vi "GetBarcode 1DResultNames.vi"(7 "ProjectName":string="Prj", 8 "error in (no error)":errorcluster, 10 "Analysis_Barcode 1D_Parameter":T2={"Barcode Search Options"={"Min Bar Width"=0.0, "Min Edge Strength"=0.0, "Min Bars"=0.0, "Skip Location Search?"=FALSE}, "Barcode Types To Search"=[enum."EAN 13", enum."Code 128", enum."Code 39"], "Barcode Grading Options"={"Calculate Grading Report"=FALSE, "Scan Width "=0.0}, "Number of Matches Requested"=1, "ROI"={"Global Rectangle"=[], "Contours"=[]}}, 11 "ROI_Name":string="ROI1") -> (0 "error out":errorcluster, 3 "ResultNames":string[](array[string]))   [LabVIEW 2019]
uses:
  Controls/Barcode 1D/Analysis_Barcode 1D_Parameter.ctl
  Controls/Barcode 1D/Analysis_Barcode 1D_Result.ctl
panel:
  out "Label.Text":string
  in  "Analysis_Barcode 1D_Result":T1 {"Barcodes"."Confidence Level" format="%.2f"; "Barcodes"."Barcode Type" items=["Reserved", "Codabar", "Code 39", "Code 93", "Code 128", "EAN 8", "EAN 13", "Interleaved 2 of 5", "MSI", "UPCA", "Pharmacode", "RSS Limited"]; "Barcodes"."Bounding Box"."y" format="%.2f"; "Barcodes"."Bounding Box"."x" format="%.2f"}
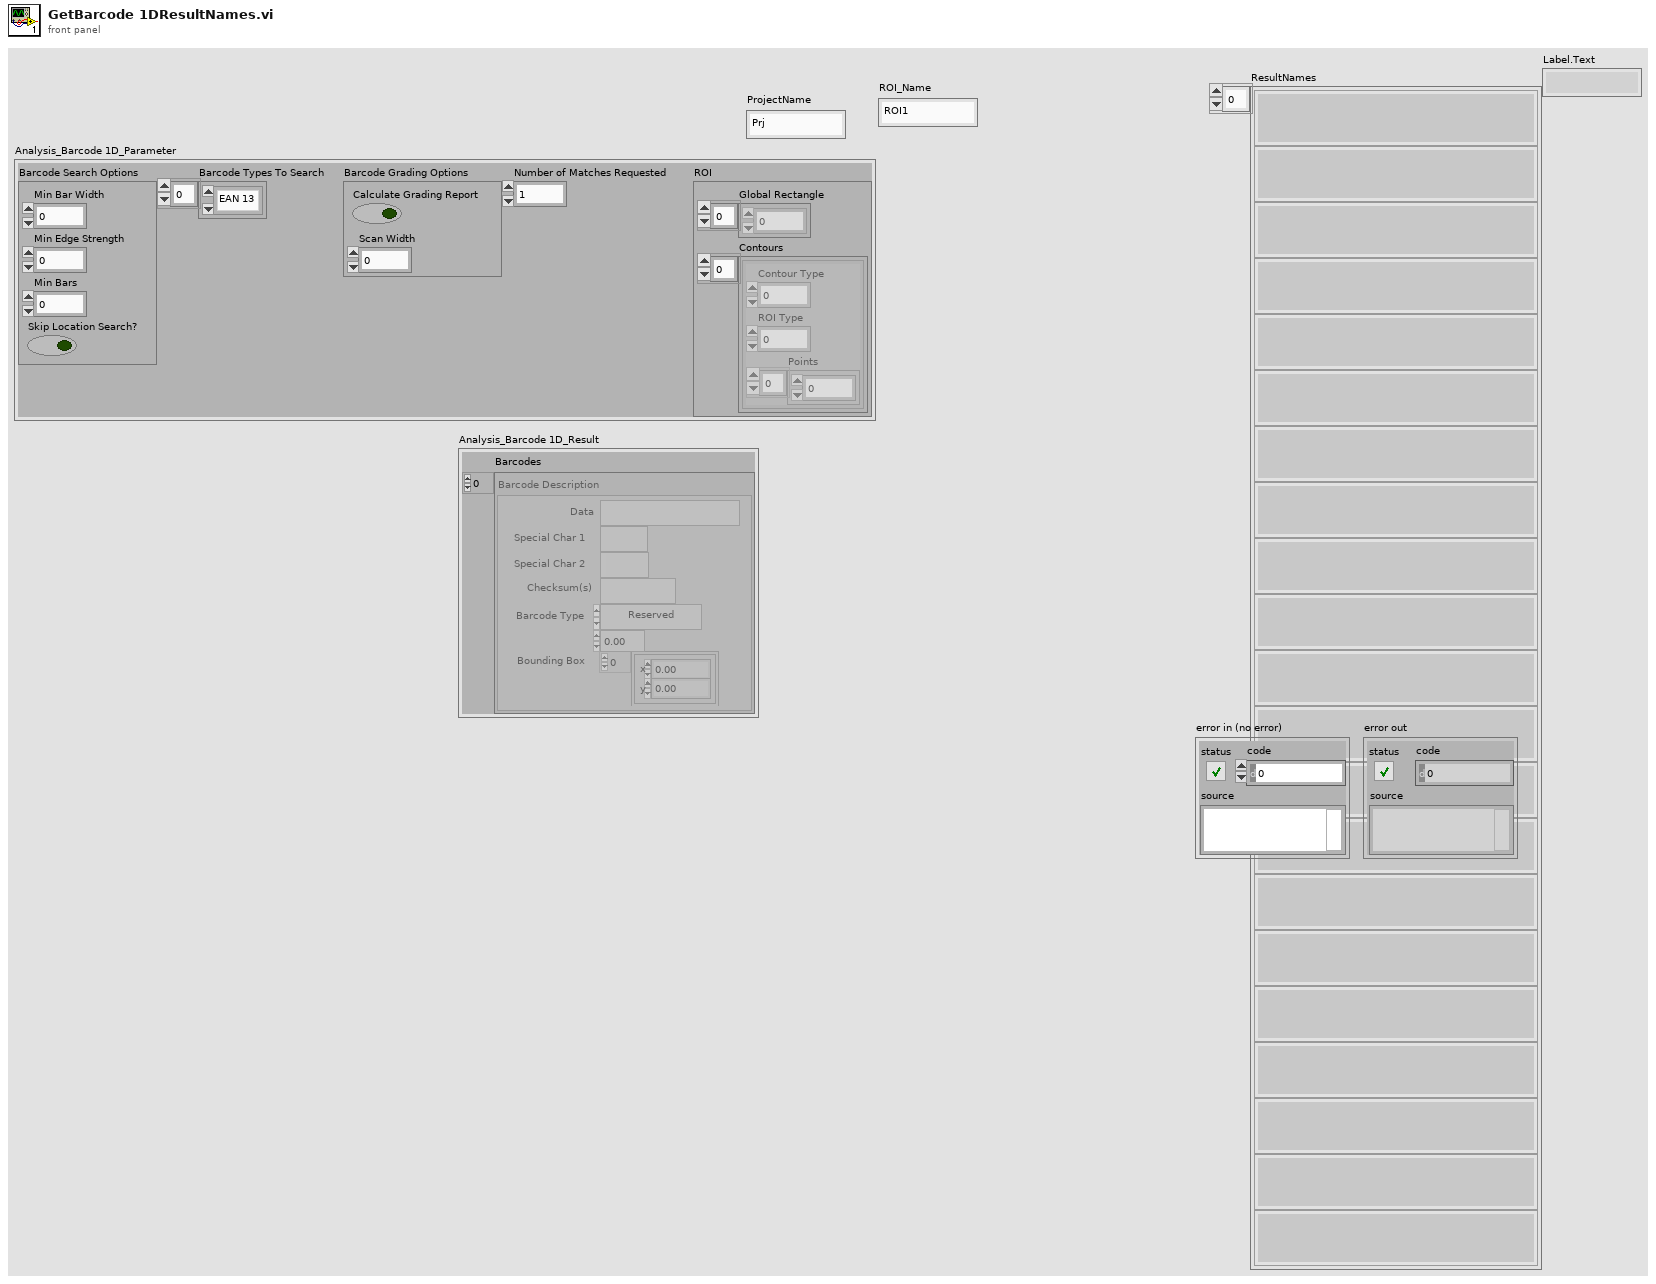
[diagram p1: front panel]
types:
  T1 = typedef "Analysis_Barcode 1D_Result.ctl" = cluster{"Barcodes":cluster{"Data":string, "Special Char 1":string, "Special Char 2":string, "Checksum(s)":string, "Barcode Type":u32, "Confidence Level":sgl, "Bounding Box":cluster{"x":sgl, "y":sgl}[]}[]}
  T2 = typedef "Analysis_Barcode 1D_Parameter.ctl" = cluster{"Barcode Search Options":cluster{"Min Bar Width":dbl, "Min Edge Strength":dbl, "Min Bars":dbl, "Skip Location Search?":bool}, "Barcode Types To Search":enum16{"Reserved", "Codabar", "Code 39", "Code 93", "Code 128", "EAN 8", "EAN 13", "Interleaved 2 of 5", "MSI", "UPCA", "Pharmacode", "RSS Limited"}[], "Barcode Grading Options":cluster{"Calculate Grading Report":bool, "Scan Width ":dbl}, "Number of Matches Requested":i32, "ROI":cluster{"Global Rectangle":i32[], "Contours":cluster{"Contour Type":u32, "ROI Type":u32, "Points":i32[]}[]}}
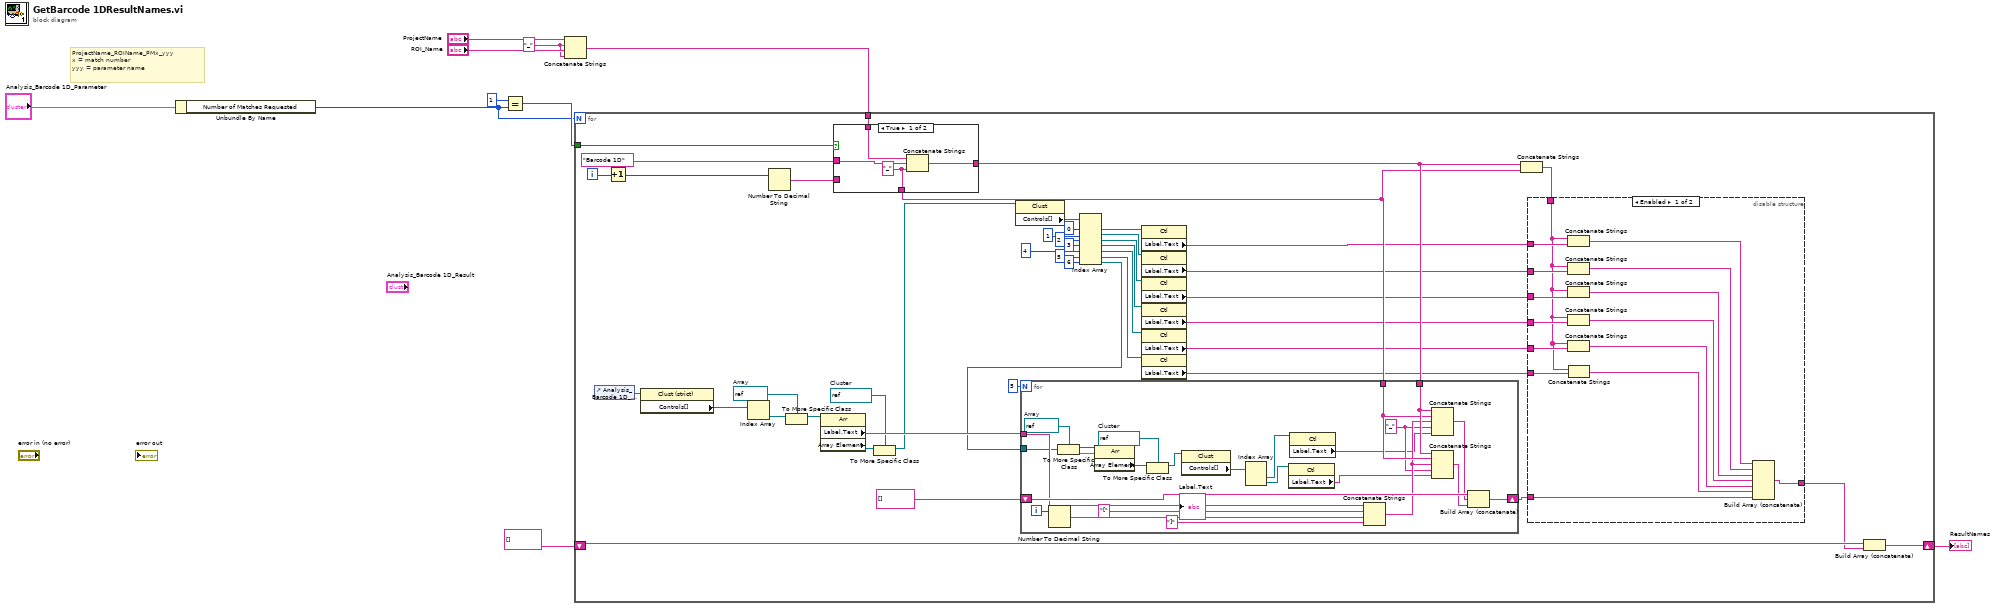
[diagram p0: block diagram]
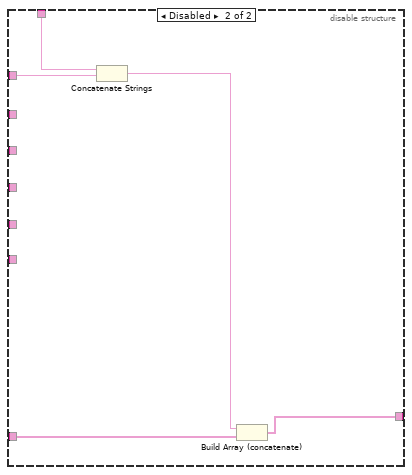
[diagram p2: hidden frame]
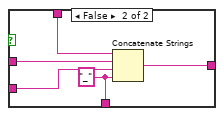
[diagram p3: hidden frame]
diagram:
  w7 = "_" ("string")
  # "ProjectName_ROIName_PMx_yyy\nx = match number\nyyy = parameter name"
  n1 = Unbundle By Name("Analysis_Barcode 1D_Parameter") -> ("Number of Matches Requested"=w1:i32)
  n2 = Equal?(x=1, y=w1) -> (x = y?=w3:bool)
  n3 = Concatenate Strings("ProjectName", w7, "ROI_Name", w7) -> (w6:string)
  n4 = for {
    N: w1 -> [_]
    tunnel: w6 -> [w53]
    shift-right: [w11] -> w4
    shift-left: string[] [] -> [w13]
    tunnel: w3 -> [w54]
    i -> [w50]
    w45 = refnum<vi> refnum  # Cluster
    w49 = refnum<vi> refnum  # Array
    n5 = control-ref of="Analysis_Barcode 1D_Result"() -> (w41:refnum<vi>)
    n6 = Increment(x=w50) -> (x+1=w55:i32)
    n7 = property class="Clust (strict)"(reference=w41) -> ("Controls[]"=w40:refnum<vi>[])  [unwired: 1 in, 2 out]
    n8 = Index Array(array=w40) -> (element=w39:refnum<vi>)  [unwired: 1 in]
    n9 = Number To Decimal String(number=w55) -> (decimal integer string=w52:string)  [unwired: 1 in]
    n10 = To More Specific Class(target class=w49, reference=w39) -> (specific class reference=w48:refnum<vi>)  [unwired: 1 in, 1 out]
    n11 = property class="Arr"(reference=w48) -> ("Label.Text"=w47:string, "Array Element"=w44:refnum<vi>)  [unwired: 1 in, 2 out]
    n12 = case shown="True" w54 {
      tunnel: w53 -> [w104 w109]
      tunnel: w52 -> [_ w107]
      tunnel: [w103 w108] -> w27
      tunnel: "Barcode 1D" ("string") -> [w102 w106]
      tunnel: [w101 w105] -> w26
      frame True {
        w101 = "_" ("string")
        n13 = Concatenate Strings(w104, w102, w101) -> (w103:string)
      }
      frame False {
        w105 = "_" ("string")
        n14 = Concatenate Strings(w109, w106, w107, w105) -> (w108:string)
      }
    }
    n15 = To More Specific Class(target class=w45, reference=w44) -> (specific class reference=w16:refnum<vi>)  [unwired: 1 in, 1 out]
    n16 = property class="Clust"(reference=w16) -> ("Controls[]"=w38:refnum<vi>[])  [unwired: 1 in, 2 out]
    n17 = Index Array(array=w38, index #1=0 ("index"), index #2=1 ("index"), index #3=2 ("index"), index #4=3 ("index"), index #5=4 ("index"), index #6=5 ("index"), index #7=6 ("index")) -> (element #1=w33:refnum<vi>, element #2=w32:refnum<vi>, element #3=w31:refnum<vi>, element #4=w30:refnum<vi>, element #5=w28:refnum<vi>, element #6=w19:refnum<vi>, element #7=w14:refnum<vi>)
    n18 = for {
      N: 5 -> [_]
      tunnel: w47 -> [w93]
      tunnel: w14 -> [w87]
      tunnel: w27 -> [w100]
      tunnel: w26 -> [w99]
      shift-right: [w95] -> w42
      shift-left: string[] [] -> [w98]
      i -> [w94]
      w82 = refnum<vi> refnum  # Cluster
      w86 = refnum<vi> refnum  # Array
      w88 = "_" ("string")
      n19 = Number To Decimal String(number=w94) -> (decimal integer string=w91:string)  [unwired: 1 in]
      n20 = To More Specific Class(target class=w86, reference=w87) -> (specific class reference=w85:refnum<vi>, error out=w84:errorcluster)  [unwired: 1 in]
      n21 = property class="Arr"(reference=w85, error in=w84) -> ("Array Element"=w83:refnum<vi>)  [unwired: 2 out]
      n22 = To More Specific Class(target class=w82, reference=w83) -> (specific class reference=w81:refnum<vi>)  [unwired: 1 in, 1 out]
      n23 = property class="Clust"(reference=w81) -> ("Controls[]"=w80:refnum<vi>[])  [unwired: 1 in, 2 out]
      n24 = Index Array(array=w80) -> (element #1=w79:refnum<vi>, element #2=w78:refnum<vi>)  [unwired: 2 in]
      n25 = property class="Ctl"(reference=w78) -> ("Label.Text"=w76:string)  [unwired: 1 in, 2 out]
      n26 = property class="Ctl"(reference=w79) -> ("Label.Text"=w77:string)  [unwired: 1 in, 2 out]
      n27 = Concatenate Strings(w93, "[" ("string"), w91, "]" ("string")) -> (w89:string)
      n28 = Concatenate Strings(w100, w99, w89, w88, w77) -> (w97:string)
      n29 = Concatenate Strings(w100, w99, w89, w88, w76) -> (w96:string)
      n30 = Build Array (concatenate)(w98, w97, w96) -> (w95:string[])
    }
    n31 = property class="Ctl"(reference=w33) -> ("Label.Text"=w25:string)  [unwired: 1 in, 2 out]
    n32 = property class="Ctl"(reference=w32) -> ("Label.Text"=w24:string)  [unwired: 1 in, 2 out]
    n33 = property class="Ctl"(reference=w31) -> ("Label.Text"=w17:string)  [unwired: 1 in, 2 out]
    n34 = property class="Ctl"(reference=w30) -> ("Label.Text"=w23:string)  [unwired: 1 in, 2 out]
    n35 = property class="Ctl"(reference=w28) -> ("Label.Text"=w22:string)  [unwired: 1 in, 2 out]
    n36 = property class="Ctl"(reference=w19) -> ("Label.Text"=w18:string)  [unwired: 1 in, 2 out]
    n37 = Concatenate Strings(w27, w26) -> (w21:string)
    n38 = disable-structure shown="Enabled" {
      disable-tunnel: w42 -> [w70 w73]
      disable-tunnel: w25 -> [w69 w75]
      disable-tunnel: w24 -> [w68 _]
      disable-tunnel: w23 -> [w67 _]
      disable-tunnel: w22 -> [w66 _]
      disable-tunnel: w21 -> [w57 w74]
      disable-tunnel: [w63 w71] -> w12
      disable-tunnel: w18 -> [w61 _]
      disable-tunnel: w17 -> [w58 _]
      frame Enabled {
        n39 = Concatenate Strings(w57, w69) -> (w65:string)
        n40 = Concatenate Strings(w57, w68) -> (w59:string)
        n41 = Concatenate Strings(w57, w58) -> (w56:string)
        n42 = Concatenate Strings(w57, w67) -> (w64:string)
        n43 = Concatenate Strings(w57, w66) -> (w62:string)
        n44 = Concatenate Strings(w57, w61) -> (w60:string)
        n45 = Build Array (concatenate)(w65, w59, w56, w64, w62, w60, w70) -> (w63:string[])
      }
      frame Disabled {
        n46 = Concatenate Strings(w74, w75) -> (w72:string)
        n47 = Build Array (concatenate)(w72, w73) -> (w71:string[])
      }
    }
    n48 = Build Array (concatenate)(w13, w12) -> (w11:string[])
  }
  "ResultNames" <- w4
